vi "Rotate and Translate Robot.vi"(9 "Robot Size (in)":cluster{"Width":dbl, "Length":dbl}, 10 "Robot Pose":cluster{"X":dbl, "Y":dbl}, 11 "Theta":dbl) -> (2 "Front Point Cursor":T1, 3 "output cluster":cluster{dbl[], dbl[]})   [LabVIEW 2025]
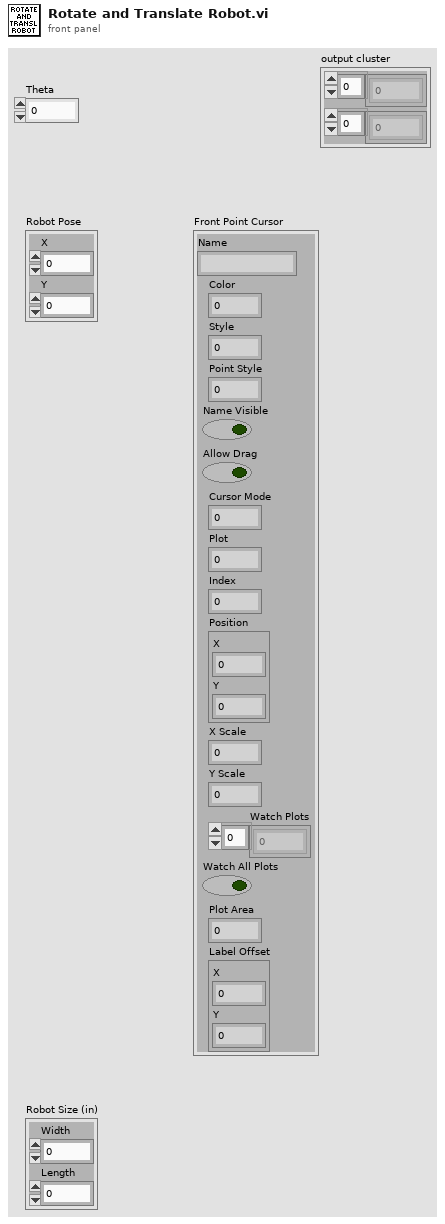
[diagram p1: front panel]
types:
  T1 = cluster{"Name":string, "Color":u32, "Style":i32, "Point Style":i32, "Name Visible":bool, "Allow Drag":bool, "Cursor Mode":u32, "Plot":i32, "Index":i32, "Position":cluster{"X":dbl, "Y":dbl}, "X Scale":u32, "Y Scale":u32, "Watch Plots":i32[], "Watch All Plots":bool, "Plot Area":i32, "Label Offset":cluster{"X":i32, "Y":i32}}
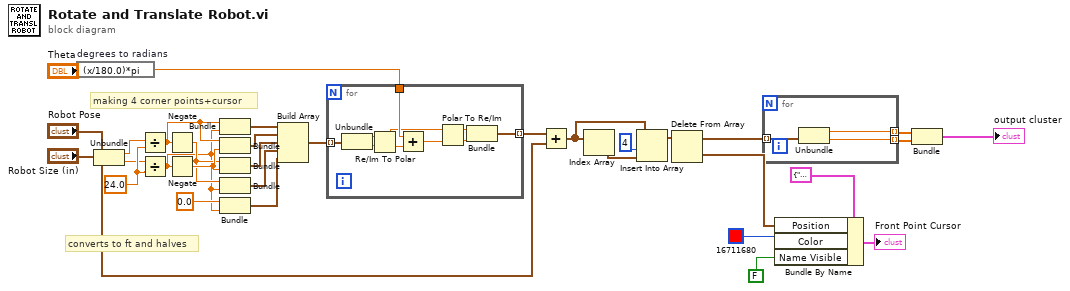
[diagram p0: block diagram]
diagram:
  w8 = 24.0 ("y")
  # "making 4 corner points+cursor"
  # "converts to ft and halves"
  n1 = expression code="(x/180.0)*pi" "degrees to radians"("Theta") -> (w21:dbl)
  n2 = Unbundle("Robot Size (in)") -> ("Width"=w6:dbl, "Length"=w7:dbl)
  n3 = Divide(x=w6, y=w8) -> (x/y=w12:dbl)
  n4 = Divide(x=w7, y=w8) -> (x/y=w10:dbl)
  n5 = Negate(x=w12) -> (-x=w13:dbl)
  n6 = Negate(x=w10) -> (-x=w14:dbl)
  n7 = Bundle(w12, w10) -> (w15:cluster{dbl, dbl})  [unwired: 1 in]
  n8 = Bundle(w12, w14) -> (w16:cluster{dbl, dbl})  [unwired: 1 in]
  n9 = Bundle(w13, w14) -> (w17:cluster{dbl, dbl})  [unwired: 1 in]
  n10 = Bundle(w13, w10) -> (w18:cluster{dbl, dbl})  [unwired: 1 in]
  n11 = Bundle(0.0, w10) -> (w19:cluster{dbl, dbl})  [unwired: 1 in]
  n12 = Build Array(w15, w16, w17, w18, w19) -> (w20:cluster{dbl, dbl}[])
  n13 = for {
    tunnel: w20 -> [w42] mode=indexing
    tunnel: w21 -> [w39]
    tunnel: [w34] -> w27 mode=indexing
    n14 = Unbundle(w42) -> (w41:dbl, w40:dbl)
    n15 = Re/Im To Polar(2:w40, 3:w41) -> (0:w38:dbl, 1:w33:dbl)
    n16 = Add(x=w39, y=w38) -> (x+y=w37:dbl)
    n17 = Polar To Re/Im(2:w37, 3:w33) -> (0:w35:dbl, 1:w36:dbl)
    n18 = Bundle(w36, w35) -> (w34:cluster{dbl, dbl})  [unwired: 1 in]
  }
  n19 = Add(x=w27, y="Robot Pose") -> (x+y=w29:cluster{dbl, dbl}[])
  n20 = Index Array(array=w29) -> (element=w31:cluster{dbl, dbl})  [unwired: 1 in]
  n21 = Insert Into Array(array=w29, index=4, new element=w31) -> (w32:cluster{dbl, dbl}[])
  n22 = Delete From Array(array=w32) -> (deleted portion=w23:cluster{dbl, dbl}, array with subset deleted=w4:cluster{dbl, dbl}[])  [unwired: 2 in]
  n23 = for {
    tunnel: w4 -> [w45] mode=indexing
    tunnel: [w44] -> w3 mode=indexing
    tunnel: [w43] -> w2 mode=indexing
    n24 = Unbundle(w45) -> (w44:dbl, w43:dbl)
  }
  n25 = Bundle By Name(cluster=T1 {"Name"="", "Color"=61192, "Style"=4, "Point Style"=6, "Name Visible"=TRUE, "Allow Drag"=TRUE, "Cursor Mode"=0, "Plot"=0, "Index"=0, "Position"={"X"=0.0, "Y"=0.0}, "X Scale"=0, "Y Scale"=0, "Watch Plots"=[], "Watch All Plots"=FALSE, "Plot Area"=0, "Label Offset"={"X"=1, "Y"=1}}, "Position"=w23, "Color"=u32 16711680, "Name Visible"=FALSE) -> (→"Front Point Cursor":T1)
  n26 = Bundle(w3, w2) -> (→"output cluster":cluster{dbl[], dbl[]})  [unwired: 1 in]
